vi "Traverse_Control_Ch_Names.vi"(1 "Traverse line":T1 {"Carrier_2 Q (l/min)" format="%#.2f"; "Row Duration (mins)" format="%#.1f"; "Row No" min=0; "Trace Gas Concentration (%)" min=0.0 format="%#_4f"; "Carrier_1 Q (l/min)" format="%#.4f"; "Start X" format="%#.2f"; "Start Y" format="%#.2f"; "Start Z" format="%#.2f"; "End X" format="%#.2f"; "End Y" format="%#.2f"; "End Z" format="%#.2f"; "Tunnel Speed" format="%#.2f"; "Averaging time (mins)" min=0.0 format="%#.2f"}, 2 "Mode":T4(ring)) -> (0 "Channel names":string[](array[string]))   [LabVIEW 2021]
uses:
  Traverse_cluster.ctl
  Spacing.ctl
  Controls/Multi_run_mode.ctl
  Globals/Extra_Commands_Global.vi
panel:
  # "X           Y          Z"
  # "Start"
  # "End"
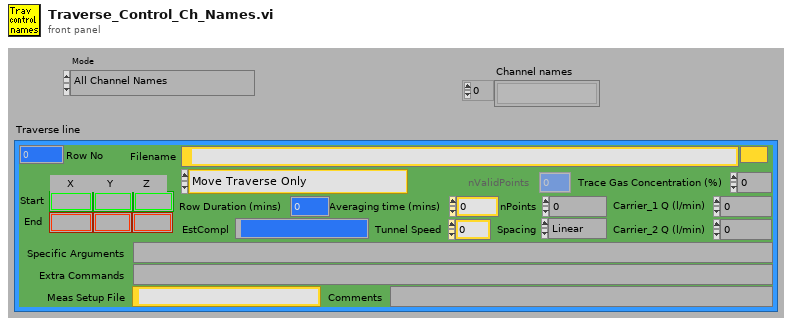
[diagram p1: front panel]
types:
  T1 = typedef "Traverse_cluster.ctl" = cluster{"Start X":sgl, "Start Y":sgl, "Start Z":sgl, "End X":sgl, "End Y":sgl, "End Z":sgl, "nPoints":i32, "Spacing":T2, "Filename":path, "Tunnel Speed":dbl, "Averaging time (mins)":dbl, "Extra Commands":string, "Carrier_1 Q (l/min)":dbl, "Carrier_2 Q (l/min)":dbl, "Trace Gas Concentration (%)":dbl, "Specific Arguments":string, "Comments":string, "Row No":i32, "Row Type Selector":T3, "EstCompl":string, "Row Duration (mins)":dbl, "nValidPoints":i32, "Meas Setup File":string}
  T2 = typedef "Spacing.ctl" = enum16{"Linear", "Log", "Gauss", "Specified", "N/A"}
  T3 = typedef "Multi_run_mode.ctl" = enum16{"Move Traverse Only", "Set Tunnel Speed Only", "Set Source Only", "Set Measurement Conditions", "Single Measurement", "Vertical Profile", "Lateral Profile", "Longitudinal Profile", "Multi-Axis Profile", "Explore Volume", "Auto Calibrate", "Meas Fast FID Bkgnd", "Check Beam Power", "Scanning Valve Measurement", "Run VI Named:", "Set ADAM Ch", "Wait (minutes)", "Send Message", "Synchronize With:", "Fall Back to this Row", "Turn Off Row Repeating", "Traverse 3D Volume", "Blank Row", "Jump to Fall Back Row"}
  T4 = enum16{"All Channel Names", "Valid Channel Names"}
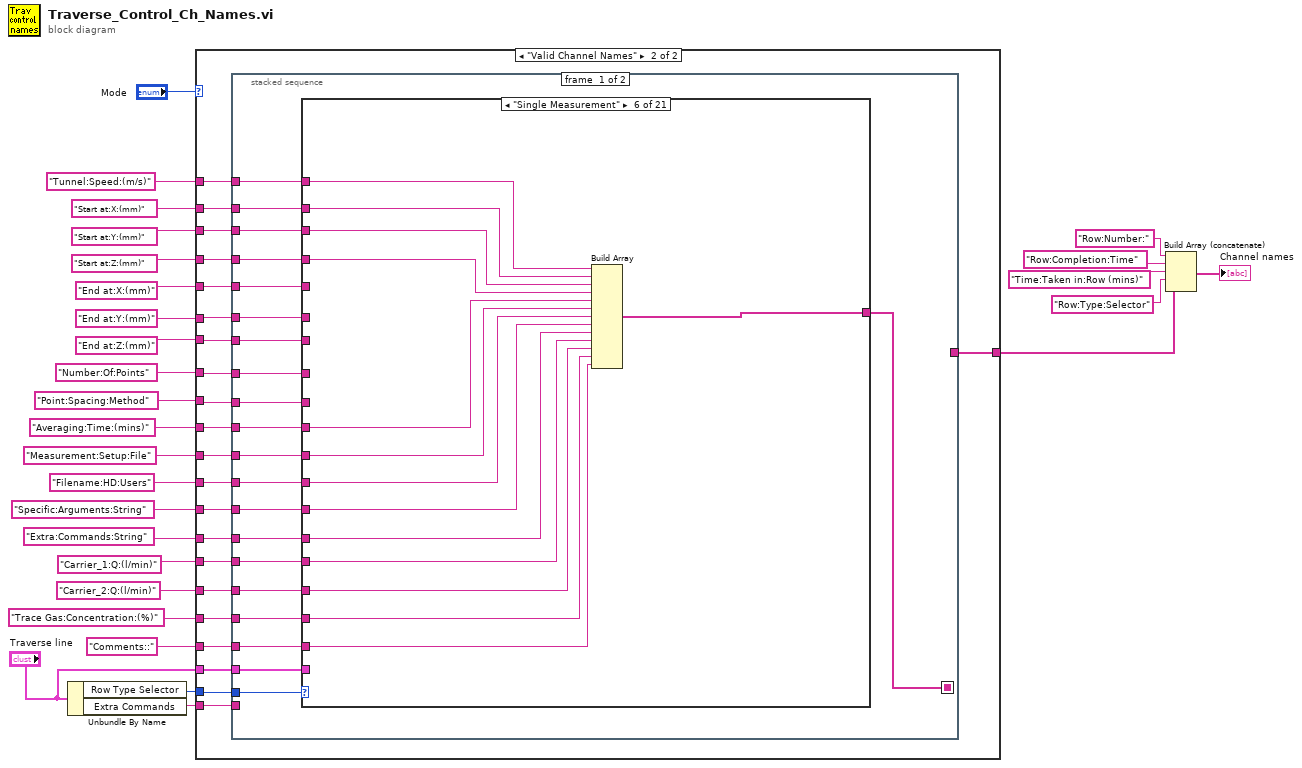
[diagram p0: block diagram]
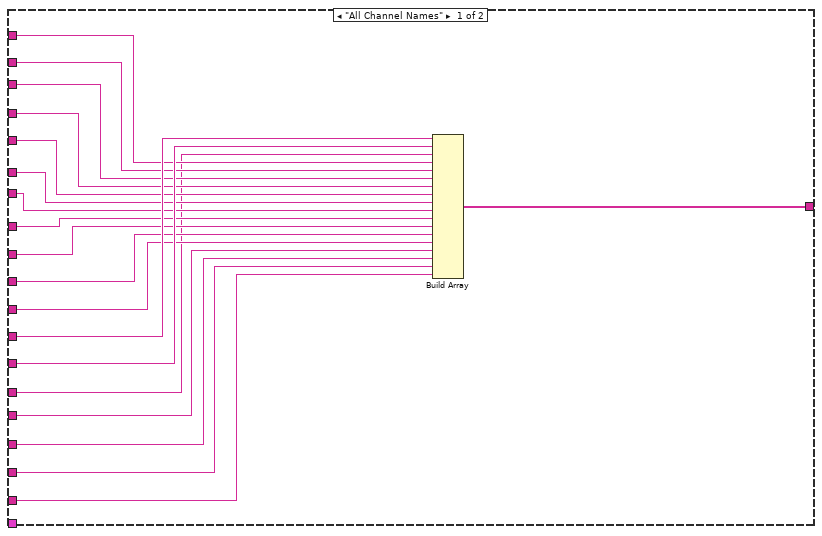
[diagram p2: hidden frame]
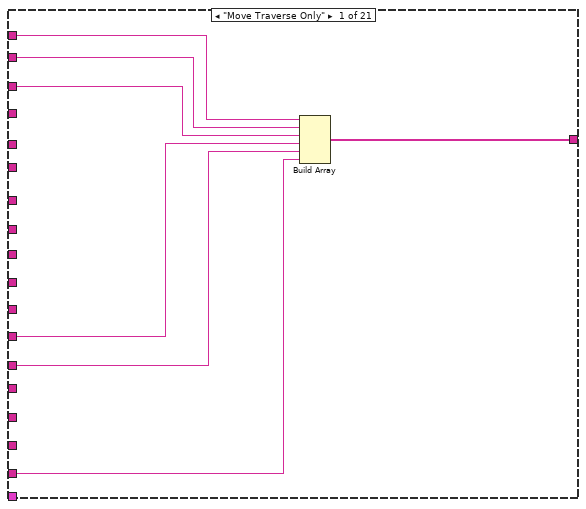
[diagram p3: hidden frame]
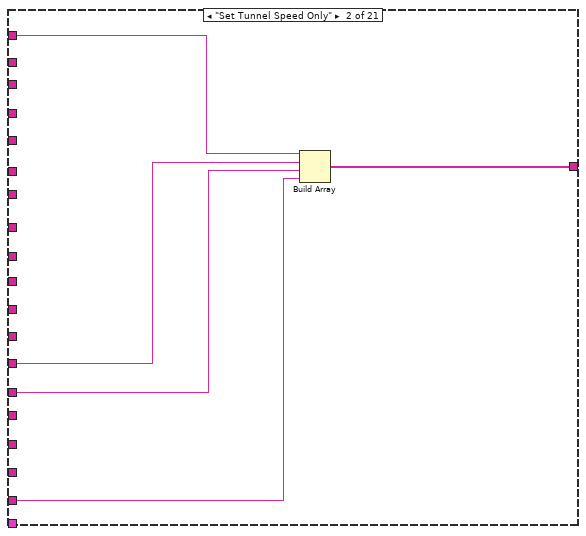
[diagram p4: hidden frame]
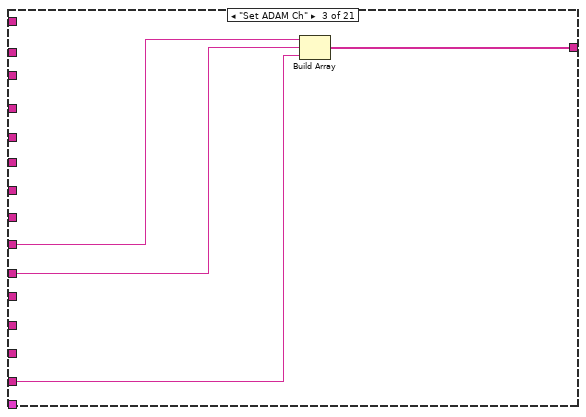
[diagram p5: hidden frame]
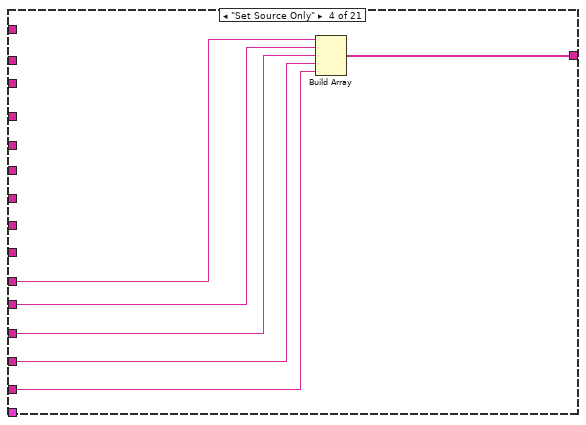
[diagram p6: hidden frame]
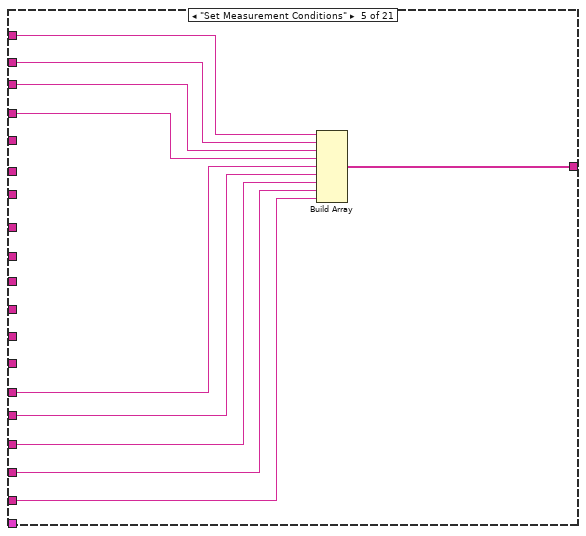
[diagram p7: hidden frame]
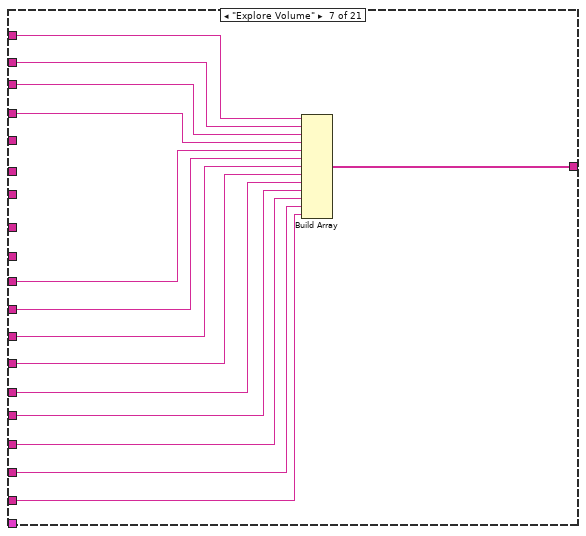
[diagram p8: hidden frame]
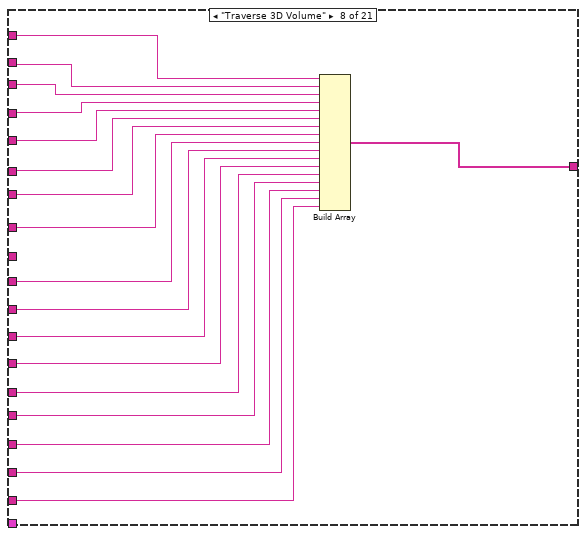
[diagram p9: hidden frame]
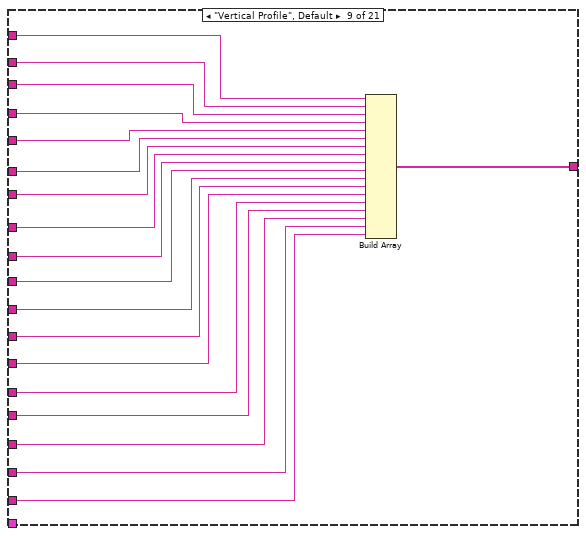
[diagram p10: hidden frame]
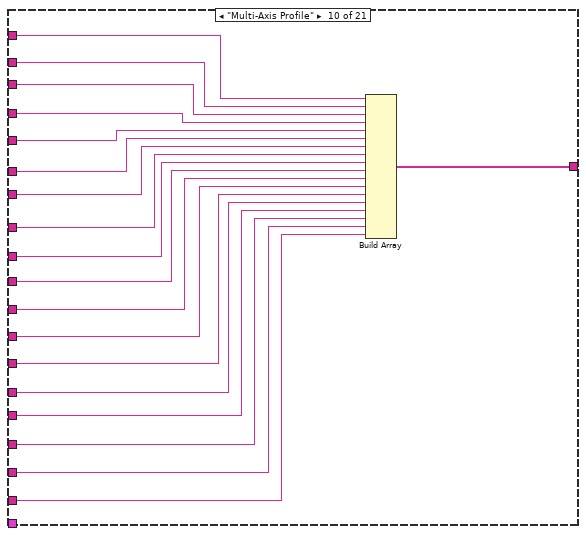
[diagram p11: hidden frame]
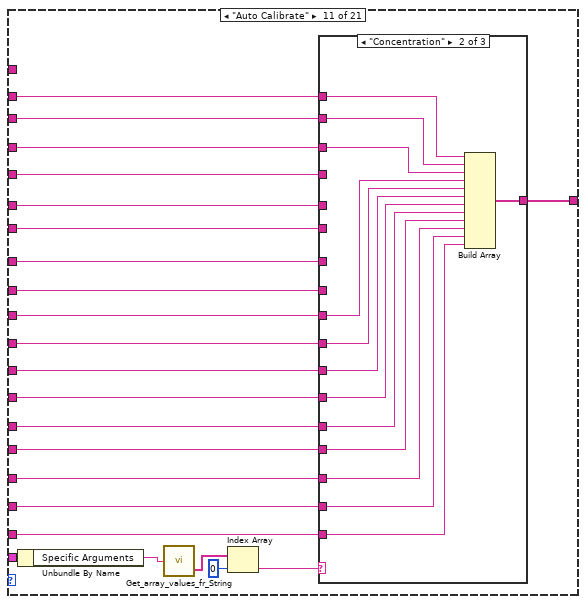
[diagram p12: hidden frame]
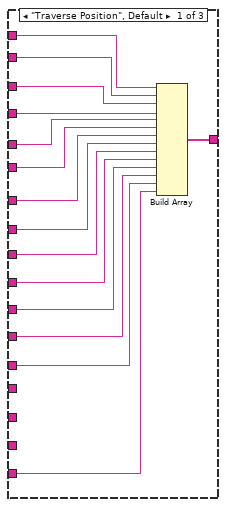
[diagram p13: hidden frame]
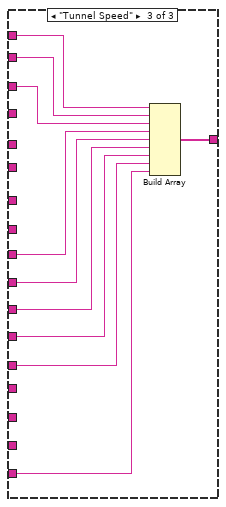
[diagram p14: hidden frame]
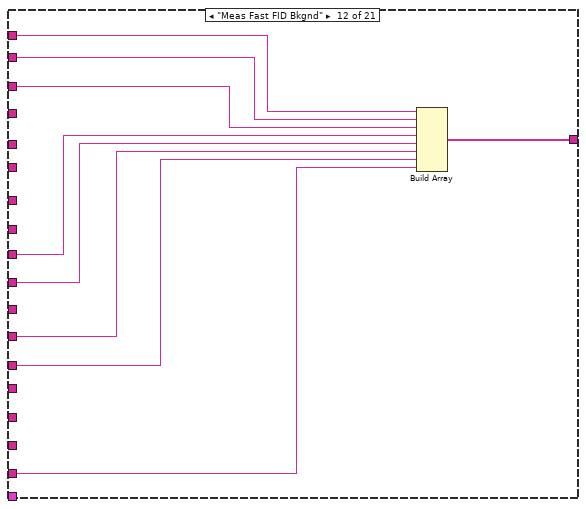
[diagram p15: hidden frame]
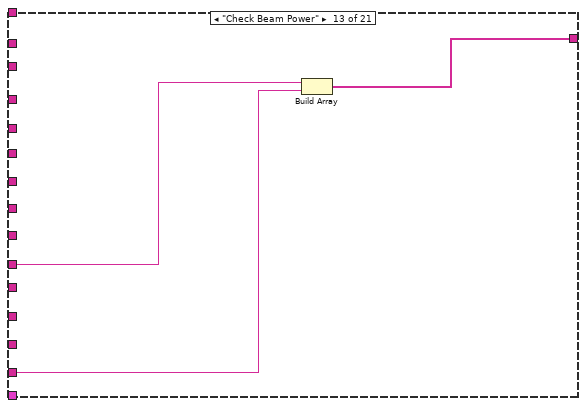
[diagram p16: hidden frame]
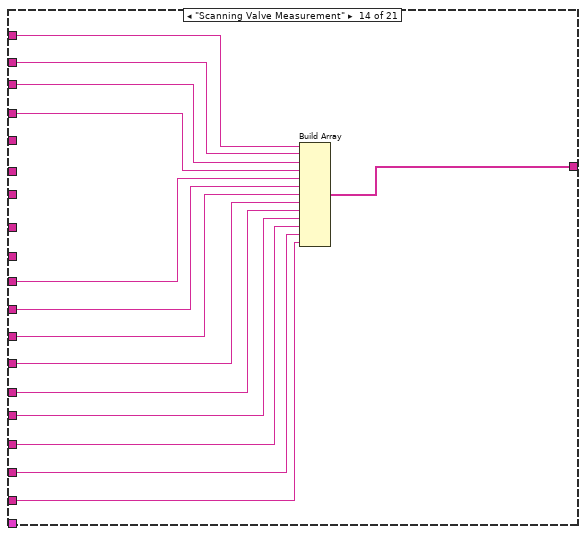
[diagram p17: hidden frame]
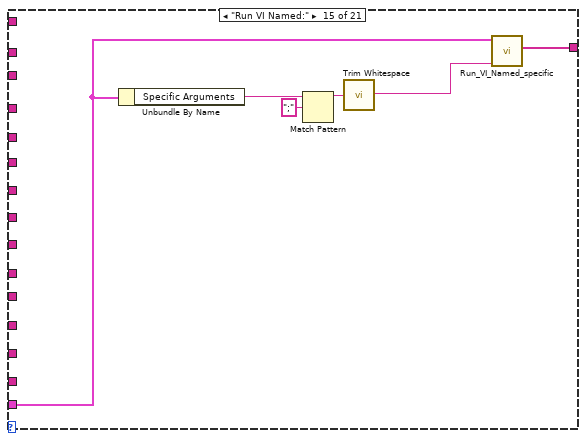
[diagram p18: hidden frame]
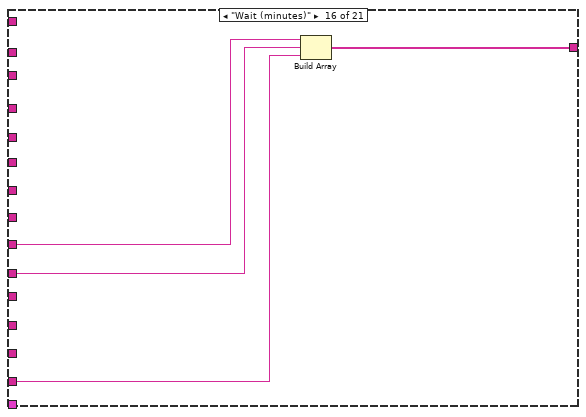
[diagram p19: hidden frame]
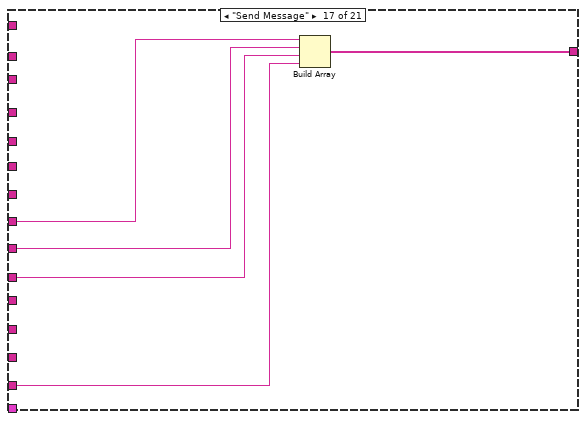
[diagram p20: hidden frame]
diagram:
  n1 = Unbundle By Name("Traverse line") -> ("Row Type Selector"=w12:T3, "Extra Commands"=w3:string)
  n2 = case shown="\"Valid Channel Names\"" "Mode" {
    tunnel: "Tunnel:Speed:(m/s)" ("Label for value") -> [w44 w68]
    tunnel: "Start at:X:(mm)" ("Label for value") -> [w43 w67]
    tunnel: "Start at:Y:(mm)" ("Label for value") -> [w42 w66]
    tunnel: "Start at:Z:(mm)" ("Label for value") -> [w41 w65]
    tunnel: "End at:X:(mm)" ("Label for value") -> [w40 w55]
    tunnel: "End at:Y:(mm)" ("Label for value") -> [w39 w54]
    tunnel: "End at:Z:(mm)" ("Label for value") -> [w38 w53]
    tunnel: "Number:Of:Points" ("Label for value") -> [w37 w52]
    tunnel: "Point:Spacing:Method" ("Label for value") -> [w36 w51]
    tunnel: "Averaging:Time:(mins)" ("Label for value") -> [w35 w57]
    tunnel: "Filename:HD:Users" ("Label for value") -> [w46 w64]
    tunnel: "Specific:Arguments:String" ("Label for value") -> [w45 w56]
    tunnel: "Extra:Commands:String" ("Label for value") -> [w29 w63]
    tunnel: "Carrier_1:Q:(l/min)" ("Label for value") -> [w34 w62]
    tunnel: "Carrier_2:Q:(l/min)" ("Label for value") -> [w33 w61]
    tunnel: "Trace Gas:Concentration:(%)" ("Label for value") -> [w32 w60]
    tunnel: "Comments::" ("Label for value") -> [w31 w59]
    tunnel: w12 -> [_ w69]
    tunnel: [w47 w58] -> w8
    tunnel: "Traverse line" -> [_ w50]
    tunnel: "Measurement:Setup:File" ("Label for value") -> [w30 w49]
    tunnel: w3 -> [_ w48]
    frame "All Channel Names" {
      n3 = Build Array(w46, w45, w29, w44, w43, w42, w41, w40, w39, w38, w37, w36, w35, w30, w34, w33, w32, w31) -> (w47:string[])
    }
    frame "Valid Channel Names" {
      n4 = stacked-sequence {
        seq-local: [w70 _] -> [_ w331]
        tunnel: w69 -> [w90 _]
        tunnel: w68 -> [w89 w329]
        tunnel: w67 -> [w88 w328]
        tunnel: w66 -> [w87 w327]
        tunnel: w65 -> [w86 w326]
        tunnel: w64 -> [w85 _]
        tunnel: w63 -> [w84 _]
        tunnel: w62 -> [w83 w318]
        tunnel: w61 -> [w82 w319]
        tunnel: w60 -> [w81 w320]
        tunnel: w59 -> [w80 _]
        tunnel: [_ w332] -> w58
        tunnel: w57 -> [w79 _]
        tunnel: w56 -> [w78 _]
        tunnel: w55 -> [w77 w325]
        tunnel: w54 -> [w76 w324]
        tunnel: w53 -> [w75 w323]
        tunnel: w52 -> [w74 w322]
        tunnel: w51 -> [w73 w321]
        tunnel: w50 -> [w72 _]
        tunnel: w49 -> [w71 _]
        tunnel: w48 -> [_ w330]
        frame #0 {
          n5 = case shown="\"Single Measurement\"" w90 {
            tunnel: w89 -> [_ w101 _ _ w121 w136 w150 w151 w187 w206 _ _ _ w293 _ _ _ _ _ _ _]
            tunnel: w88 -> [w97 _ _ _ w120 w135 w149 w152 w186 w205 w229 w272 _ w292 _ _ _ _ _ _ _]
            tunnel: w87 -> [w96 _ _ _ w119 w134 w148 w153 w185 w204 w228 w271 _ w291 _ _ _ _ _ _ _]
            tunnel: w86 -> [w95 _ _ _ w118 w133 w147 w154 w184 w203 w227 w270 _ w290 _ _ _ _ _ _ _]
            tunnel: w85 -> [_ _ _ _ _ w130 w144 w166 w176 w195 w220 _ _ w287 _ _ w304 _ _ _ _]
            tunnel: w84 -> [w93 w100 w103 w111 w117 w125 w139 w161 w174 w193 w218 w274 w277 w285 _ w301 w306 _ _ _ _]
            tunnel: w83 -> [_ _ _ w110 w116 w129 w143 w165 w173 w192 w209 _ _ w284 _ _ _ _ _ _ _]
            tunnel: w82 -> [_ _ _ w109 w115 w128 w142 w164 w172 w191 w208 _ _ w283 _ _ _ _ _ _ _]
            tunnel: w81 -> [_ _ _ w108 w114 w127 w141 w163 w171 w190 w207 _ _ w282 _ _ _ _ _ _ _]
            tunnel: w80 -> [w92 w99 w105 w107 w113 w126 w140 w162 w170 w189 w217 w275 w278 w281 _ w300 w305 w309 w312 w314 w317]
            tunnel: [w94 w102 w106 w112 w122 w132 w146 w168 w183 w202 w226 w276 w279 w289 w294 w303 w308 w311 w313 w315 w316] -> w70
            tunnel: w79 -> [_ _ _ _ _ w131 w145 w167 w177 w196 w214 w269 _ w288 _ _ _ _ _ _ _]
            tunnel: w78 -> [w91 w98 w104 _ _ w123 w138 w160 w175 w194 w219 w273 _ w286 _ w302 w307 w310 _ _ _]
            tunnel: w77 -> [_ _ _ _ _ _ _ w155 w182 w201 w225 _ _ _ _ _ _ _ _ _ _]
            tunnel: w76 -> [_ _ _ _ _ _ _ w156 w181 w200 w224 _ _ _ _ _ _ _ _ _ _]
            tunnel: w75 -> [_ _ _ _ _ _ _ w157 w180 w199 w223 _ _ _ _ _ _ _ _ _ _]
            tunnel: w74 -> [_ _ _ _ _ _ _ w158 w179 w198 w222 _ _ _ _ _ _ _ _ _ _]
            tunnel: w73 -> [_ _ _ _ _ _ _ _ w178 w197 w221 _ _ _ _ _ _ _ _ _ _]
            tunnel: w72 -> [_ _ _ _ _ _ _ _ _ _ w216 _ _ _ w295 _ _ _ _ _ _]
            tunnel: w71 -> [_ _ _ _ _ w124 w137 w159 w169 w188 w215 w268 _ w280 _ _ _ _ _ _ _]
            frame "Move Traverse Only" {
              n6 = Build Array(w97, w96, w95, w91, w93, w92) -> (w94:string[])
            }
            frame "Set Tunnel Speed Only" {
              n7 = Build Array(w101, w98, w100, w99) -> (w102:string[])
            }
            frame "Set ADAM Ch" {
              n8 = Build Array(w104, w103, w105) -> (w106:string[])
            }
            frame "Set Source Only" {
              n9 = Build Array(w111, w110, w109, w108, w107) -> (w112:string[])
            }
            frame "Set Measurement Conditions" {
              n10 = Build Array(w121, w120, w119, w118, w117, w116, w115, w114, w113) -> (w122:string[])
            }
            frame "Single Measurement" {
              n11 = Build Array(w136, w135, w134, w133, w131, w124, w130, w123, w125, w129, w128, w127, w126) -> (w132:string[])
            }
            frame "Explore Volume" {
              n12 = Build Array(w150, w149, w148, w147, w145, w137, w144, w138, w139, w143, w142, w141, w140) -> (w146:string[])
            }
            frame "Traverse 3D Volume" {
              n13 = Build Array(w151, w152, w153, w154, w155, w156, w157, w158, w167, w159, w166, w160, w161, w165, w164, w163, w162) -> (w168:string[])
            }
            frame "Vertical Profile", Default {
              n14 = Build Array(w187, w186, w185, w184, w182, w181, w180, w179, w178, w177, w169, w176, w175, w174, w173, w172, w171, w170) -> (w183:string[])
            }
            frame "Multi-Axis Profile" {
              n15 = Build Array(w206, w205, w204, w203, w201, w200, w199, w198, w197, w196, w188, w195, w194, w193, w192, w191, w190, w189) -> (w202:string[])
            }
            frame "Auto Calibrate" {
              n16 = Unbundle By Name(w216) -> ("Specific Arguments"=w213:string)
              n17 = call "Get_array_values_fr_String.vi"("String Value"=w213) -> ("String array"=w211:string[])  [unwired: 1 out]
              n18 = Index Array(array=w211, index=0 ("Index")) -> (element=w210:string)
              n19 = case shown="\"Concentration\"" w210 {
                tunnel: w229 -> [w244 w257 w267]
                tunnel: w228 -> [w243 w256 w266]
                tunnel: w227 -> [w242 w255 w265]
                tunnel: [w241 w254 w264] -> w226
                tunnel: w225 -> [w240 _ _]
                tunnel: w224 -> [w239 _ _]
                tunnel: w223 -> [w238 _ _]
                tunnel: w222 -> [w237 _ _]
                tunnel: w221 -> [w236 _ _]
                tunnel: w220 -> [w235 w253 w263]
                tunnel: w219 -> [w234 w252 w262]
                tunnel: w218 -> [w233 w251 w261]
                tunnel: w217 -> [w232 w245 w260]
                tunnel: w215 -> [w231 w250 w259]
                tunnel: w214 -> [w230 w249 w258]
                tunnel: w209 -> [_ w248 _]
                tunnel: w208 -> [_ w247 _]
                tunnel: w207 -> [_ w246 _]
                frame "Traverse Position", Default {
                  n20 = Build Array(w244, w243, w242, w240, w239, w238, w237, w236, w230, w231, w235, w234, w233, w232) -> (w241:string[])
                }
                frame "Concentration" {
                  n21 = Build Array(w257, w256, w255, w249, w250, w253, w252, w251, w248, w247, w246, w245) -> (w254:string[])
                }
                frame "Tunnel Speed" {
                  n22 = Build Array(w267, w266, w265, w258, w259, w263, w262, w261, w260) -> (w264:string[])
                }
              }
            }
            frame "Meas Fast FID Bkgnd" {
              n23 = Build Array(w272, w271, w270, w269, w268, w273, w274, w275) -> (w276:string[])
            }
            frame "Check Beam Power" {
              n24 = Build Array(w277, w278) -> (w279:string[])
            }
            frame "Scanning Valve Measurement" {
              n25 = Build Array(w293, w292, w291, w290, w288, w280, w287, w286, w285, w284, w283, w282, w281) -> (w289:string[])
            }
            frame "Run VI Named:" {
              n26 = Unbundle By Name(w295) -> ("Specific Arguments"=w297:string)
              n27 = Match Pattern(string=w297, regular expression=";") -> (before substring=w299:string)  [unwired: 4 out]
              n28 = call <vilib>:"Trim Whitespace.vi"("string"=w299) -> ("trimmed string"=w296:string)  [unwired: 1 in]
              n29 = call "Run_VI_Named_specific.vi"("Run VI Named String"=w296, "Multi Run Row"=w295) -> ("Channel Names"=w294:string[])  [unwired: 1 in, 8 out]
            }
            frame "Wait (minutes)" {
              n30 = Build Array(w302, w301, w300) -> (w303:string[])
            }
            frame "Send Message" {
              n31 = Build Array(w304, w307, w306, w305) -> (w308:string[])
            }
            frame "Synchronize With:" {
              n32 = Build Array(w310, w309) -> (w311:string[])
            }
            frame "Fall Back to this Row" {
              n33 = Build Array(w312) -> (w313:string[])
            }
            frame "Blank Row" {
              n34 = Build Array(w314) -> (w315:string[])
            }
            frame "Turn Off Row Repeating" {
              n35 = Build Array(w317) -> (w316:string[])
            }
          }
        }
        frame #1 {
          n36 = Empty String/Path?(string/path=w330) -> (empty?=w333:bool)
          n37 = case shown="False" w333 {
            tunnel: [w334 w392] -> w332
            tunnel: w331 -> [w336 w392]
            tunnel: w330 -> [w340 _]
            tunnel: w329 -> [w347 _]
            tunnel: w328 -> [w359 _]
            tunnel: w327 -> [w358 _]
            tunnel: w326 -> [w357 _]
            tunnel: w325 -> [w356 _]
            tunnel: w324 -> [w355 _]
            tunnel: w323 -> [w354 _]
            tunnel: w322 -> [w353 _]
            tunnel: w321 -> [w352 _]
            tunnel: w320 -> [w345 _]
            tunnel: w319 -> [w344 _]
            tunnel: w318 -> [w343 _]
            frame False {
              n38 = global read "Extra_Commands_Global.vi" "Skip Traverse Position Demand"() -> (w360:string)
              n39 = global read "Extra_Commands_Global.vi" "Skip Tunnel Speed Demand"() -> (w349:string)
              n40 = Match Pattern(string=w340, regular expression=w360) -> (offset past match=w361:i32)  [unwired: 4 out]
              n41 = global read "Extra_Commands_Global.vi" "Skip Source Demand"() -> (w339:string)
              n42 = Match Pattern(string=w340, regular expression=w349) -> (offset past match=w350:i32)  [unwired: 4 out]
              n43 = Greater Than 0?(x=w361) -> (x > 0?=w351:bool)
              n44 = case shown="True" w351 {
                tunnel: w359 -> [_ w391]
                tunnel: w358 -> [_ w390]
                tunnel: w357 -> [_ w389]
                tunnel: w356 -> [_ w388]
                tunnel: w355 -> [_ w387]
                tunnel: w354 -> [_ w386]
                tunnel: w353 -> [_ w385]
                tunnel: w352 -> [_ w384]
                tunnel: [string[] [] w383] -> w346
                frame False {
                }
                frame True {
                  n45 = Build Array(w391, w390, w389, w388, w387, w386, w385, w384) -> (w383:string[])
                }
              }
              n46 = Greater Than 0?(x=w350) -> (x > 0?=w348:bool)
              n47 = case shown="True" w348 {
                tunnel: w347 -> [_ w381]
                tunnel: w346 -> [w378 w380]
                tunnel: [w378 w379] -> w342
                frame False {
                }
                frame True {
                  n48 = Build Array (concatenate)(w381, w380) -> (w379:string[])
                }
              }
              n49 = Match Pattern(string=w340, regular expression=w339) -> (offset past match=w341:i32)  [unwired: 4 out]
              n50 = Greater Than 0?(x=w341) -> (x > 0?=w338:bool)
              n51 = case shown="True" w338 {
                tunnel: w343 -> [_ w377]
                tunnel: w344 -> [_ w376]
                tunnel: w345 -> [_ w375]
                tunnel: [w372 w374] -> w337
                tunnel: w342 -> [w372 w373]
                frame False {
                }
                frame True {
                  n52 = Build Array (concatenate)(w373, w377, w376, w375) -> (w374:string[])
                }
              }
              n53 = for {
                shift-right: [w362] -> w334
                shift-left: string[] [] -> [w364]
                tunnel: w337 -> [w367]
                tunnel: w336 -> [w363] mode=indexing
                n54 = Search 1D Array(1D array=w367, element=w363) -> (index of element=w366:i32)  [unwired: 1 out]
                n55 = Less Than 0?(x=w366) -> (x < 0?=w365:bool)
                n56 = case shown="True" w365 {
                  tunnel: w364 -> [w368 w371]
                  tunnel: w363 -> [_ w370]
                  tunnel: [w368 w369] -> w362
                  frame False {
                  }
                  frame True {
                    n57 = Build Array (concatenate)(w371, w370) -> (w369:string[])
                  }
                }
              }
            }
            frame True {
            }
          }
        }
      }
    }
  }
  n58 = Build Array (concatenate)("Row:Number:" ("Label for value"), "Row:Completion:Time" ("Label for value"), "Time:Taken in:Row (mins)" ("Label for value"), "Row:Type:Selector" ("Label for value"), w8) -> (→"Channel names":string[])
